vi "Select Controller.vi"(6 "Type":enum16{"PID", "Industrial"}(ring), 10 "CD Path":string, 11 "NIVS.System Definition Root":refnum<k24>) -> (1 "Cancelled?":bool, 2 "IP Address":string="Targets/Controller/Custom Devices/Communication Example", 3 "Custom Device Path Out":string="Targets/Controller/Custom Devices/Communication Example")   [LabVIEW 2019, in "Control Workspace Object.lvlib"]
uses:
  NationalInstruments.VeriStand.SystemStorage
  Control Workspace Object.lvlib
panel:
  in  "Cancel":bool
  in  "Select":bool
  in  "Custom Device Path":string(tree)
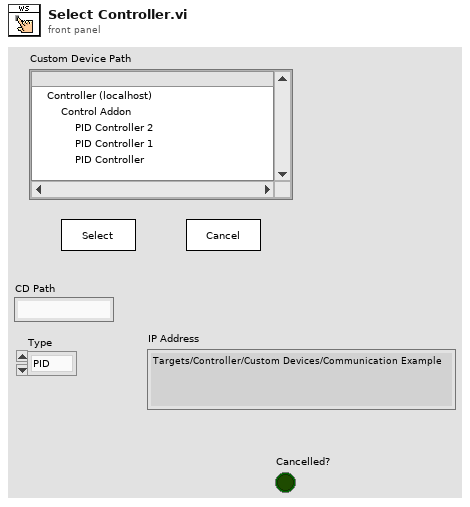
[diagram p1: front panel]
types:
  T1 = enum8{"Enabled", "Disabled", "Disabled and Grayed Out"}
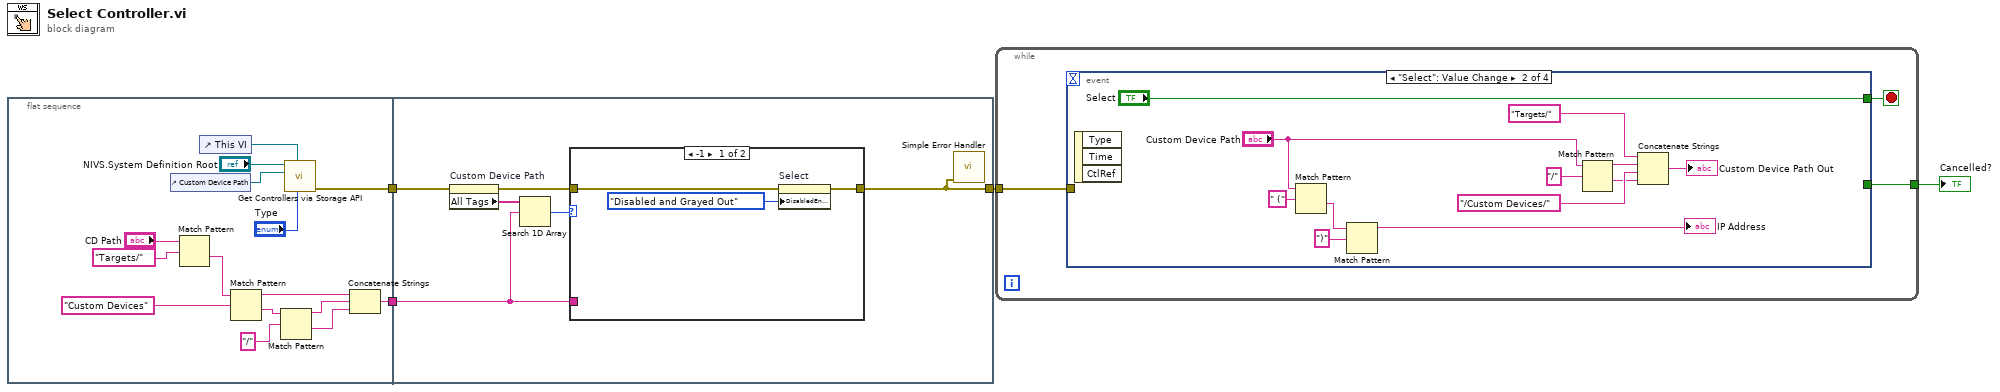
[diagram p0: block diagram]
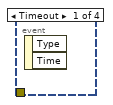
[diagram p2: hidden frame]
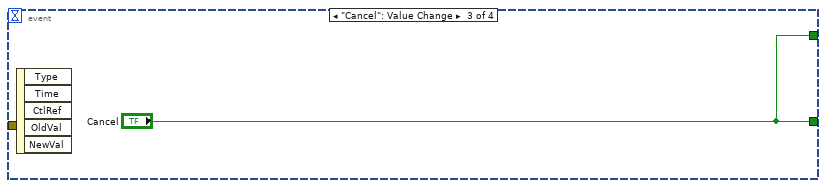
[diagram p3: hidden frame]
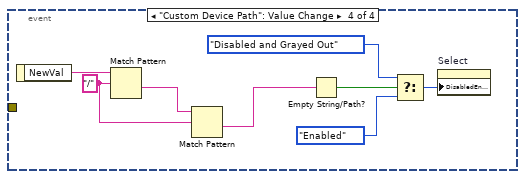
[diagram p4: hidden frame]
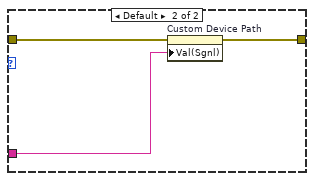
[diagram p5: hidden frame]
diagram:
  n1 = flat-sequence {
    tunnel: [w17] -> w3
    tunnel: [w10] -> w1
    tunnel: [w25] -> w4
    tunnel: w3 -> [w24]
    tunnel: w1 -> [w21]
    frame #0 {
      n2 = control-ref of="Custom Device Path"() -> (w18:refnum<vi>)
      n3 = Match Pattern(string="CD Path", regular expression="Targets/") -> (after substring=w13:string)  [unwired: 1 in, 3 out]
      n4 = control-ref of="This VI"() -> (w16:refnum<vi>)
      n5 = Match Pattern(string=w13, regular expression="Custom Devices") -> (before substring=w15:string, after substring=w9:string)  [unwired: 1 in, 2 out]
      n6 = Match Pattern(string=w9, regular expression="/") -> (before substring=w7:string, after substring=w6:string)  [unwired: 1 in, 2 out]
      n7 = call "Get Controllers via Storage API.vi"("Action"="Type", "VI reference (current VI)"=w16, "Tree"=w18, "NIVS.System Definition Root"="NIVS.System Definition Root") -> ("error out"=w17:errorcluster)  [unwired: 6 in, 1 out]
      n8 = Concatenate Strings(w15, w7, w6) -> (w10:string)
    }
    frame #1 {
      n9 = property on="Custom Device Path" class="Tree (strict)"(error in=w24) -> (error out=w23:errorcluster, "All Tags"=w22:string[])  [unwired: 1 in, 1 out]
      n10 = Search 1D Array(1D array=w22, element=w21) -> (index of element=w20:i32)  [unwired: 1 in]
      n11 = case shown="-1" w20 {
        tunnel: [w28 w31] -> w25
        tunnel: w23 -> [w27 w30]
        tunnel: w21 -> [_ w29]
        frame -1 {
          n12 = property on="Select" class="Bool"(error in=w27, "DisabledEnum"=T1."Disabled and Grayed Out" ("Disabled")) -> (error out=w28:errorcluster)  [unwired: 1 in, 1 out]
        }
        frame Default {
          n13 = property on="Custom Device Path" class="Tree (strict)"(error in=w30, "Val(Sgnl)"=w29) -> (error out=w31:errorcluster)  [unwired: 1 in, 1 out]
        }
      }
      n14 = call <vilib>:"Simple Error Handler.vi"("error in (no error)"=w25) -> ()  [unwired: 4 in, 5 out]
    }
  }
  n15 = while {
    tunnel: w4 -> [w34]
    tunnel: [w32] -> w2
    stop <- w33 stop-if-true
    n16 = event shown="[1] \"Select\": Value Change" {
      selector: _ -> [_ _ _ _]
      dyn-events: _ -> [_ _ _ _]
      timeout: _ -> [_ _ _ _]
      tunnel: w34 -> [_ _ _ _]
      tunnel: [_ "Select" "Cancel" _] -> w33
      tunnel: [_ _ "Cancel" _] -> w32
      event Timeout {
        n17 = event-data() -> ()  [unwired: 1 in, 2 out]
      }
      event "Select": Value Change {
        n18 = event-data() -> ()  [unwired: 1 in, 3 out]
        n19 = Match Pattern(string="Custom Device Path", regular expression=" (") -> (after substring=w37:string)  [unwired: 1 in, 3 out]
        n20 = Match Pattern(string=w37, regular expression=")") -> (before substring=→"IP Address":string)  [unwired: 1 in, 3 out]
        n21 = Match Pattern(string="Custom Device Path", regular expression="/") -> (before substring=w44:string, after substring=w42:string)  [unwired: 1 in, 2 out]
        n22 = Concatenate Strings("Targets/" ("string"), w44, "/Custom Devices/" ("string"), w42) -> (→"Custom Device Path Out":string)
      }
      event "Cancel": Value Change {
        n23 = event-data() -> ()  [unwired: 1 in, 5 out]
      }
      event "Custom Device Path": Value Change {
        w50 = "/" ("regular expression")
        n24 = event-data() -> ("NewVal"=w55:string)  [unwired: 1 in]
        n25 = Match Pattern(string=w55, regular expression=w50) -> (after substring=w49:string)  [unwired: 1 in, 3 out]
        n26 = Match Pattern(string=w49, regular expression=w50) -> (after substring=w48:string)  [unwired: 1 in, 3 out]
        n27 = Empty String/Path?(string/path=w48) -> (empty?=w54:bool)
        n28 = Select(t=T1."Disabled and Grayed Out" ("Disabled"), s=w54, f=T1."Enabled" ("Disabled")) -> (s? t:f=w51:T1)
        n29 = property on="Select" class="Bool"("DisabledEnum"=w51) -> ()  [unwired: 2 in, 2 out]
      }
    }
  }
  "Cancelled?" <- w2
